vi "ErrorHandlerLabel.vi"(11 "Sorted Errors":T2(array[cluster])) -> (3 "Error Cluster Out":T1(array[cluster]))   [LabVIEW 2015]
uses:
  GlobalBoardIDs.vi
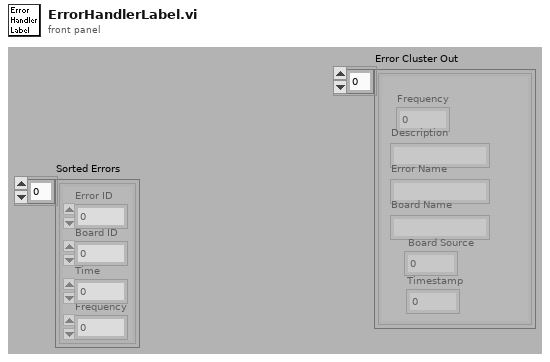
[diagram p1: front panel]
types:
  T1 = cluster{"Frequency":dbl, "Description":string, "Error Name":string, "Board Name":string, " Board Source":dbl, "Timestamp":dbl}[]
  T2 = cluster{"Error ID":i32, "Board ID":i32, "Time":u32, "Frequency":i32}[]
  T3 = cluster{"Frequency":i32, "Description":string, "Error Name":string, "String":string, "Board ID":i32, "Time":u32}
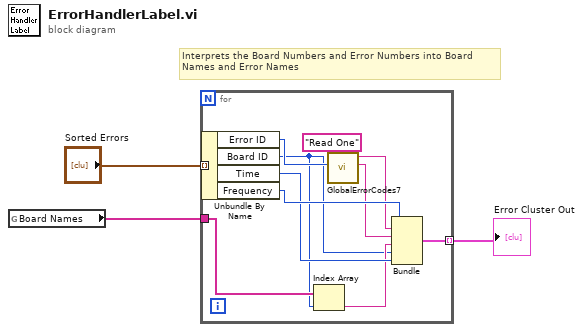
[diagram p0: block diagram]
diagram:
  # "Interprets the Board Numbers and Error Numbers into Board\nNames and Error Names"
  n1 = global read "GlobalBoardIDs.vi" "Board Names"() -> (w2:string[])
  n2 = for {
    tunnel: "Sorted Errors" -> [w13] mode=indexing
    tunnel: w2 -> [w10]
    tunnel: [w8] -> w1 mode=indexing
    (unwired) "Read One" ("Function select")
    n3 = Unbundle By Name(w13) -> ("Error ID"=w5:i32, "Board ID"=w4:i32, "Time"=w11:u32, "Frequency"=w12:i32)
    n4 = Index Array(array=w10, index=w4) -> (element=w9:string)
    n5 = call "GlobalErrorCodes7.vi"("Element #"=w5) -> ("Error Name"=w7:string, "Description"=w6:string)  [unwired: 3 in, 2 out]
    n6 = Bundle("Frequency"=w12, "Description"=w6, "Error Name"=w7, "String"=w9, "Board ID"=w4, "Time"=w11) -> (w8:T3)  [unwired: 1 in]
  }
  "Error Cluster Out" <- w1
